vi "p4.3.vi"() -> ()   [LabVIEW 2020]
uses:
  <vilib>/Analysis/2dsp.llb/Upsample (DBL).vi
  <vilib>/Analysis/NI_AALBase.lvlib
  <vilib>/Analysis/NI_AALPro.lvlib
panel:
  out "FFT(Expansor L=3)":dbl[](graph)
  out "FFT(Expansor L=2)":dbl[](graph)
  out "FFT(original)":dbl[](graph)
  in  "L =3":i32=1
  out "Expansor L=3":dbl[](graph)
  out "Expansor L=2":dbl[](graph)
  in  "L=2":i32=1
  out "cos(0,0.3pi) + cos(0,0.4pi) - Original":dbl[](graph)
  in  "Frecuencia cos(0,4pi)":dbl=0.0078125 format="%0.4e"
  out "cos(0,0.4pi)":dbl[](graph)
  out "cos(0,0.3pi)":dbl[](graph)
  in  "Frecuencia cos(0,3pi)":dbl=0.0078125 format="%0.4e"
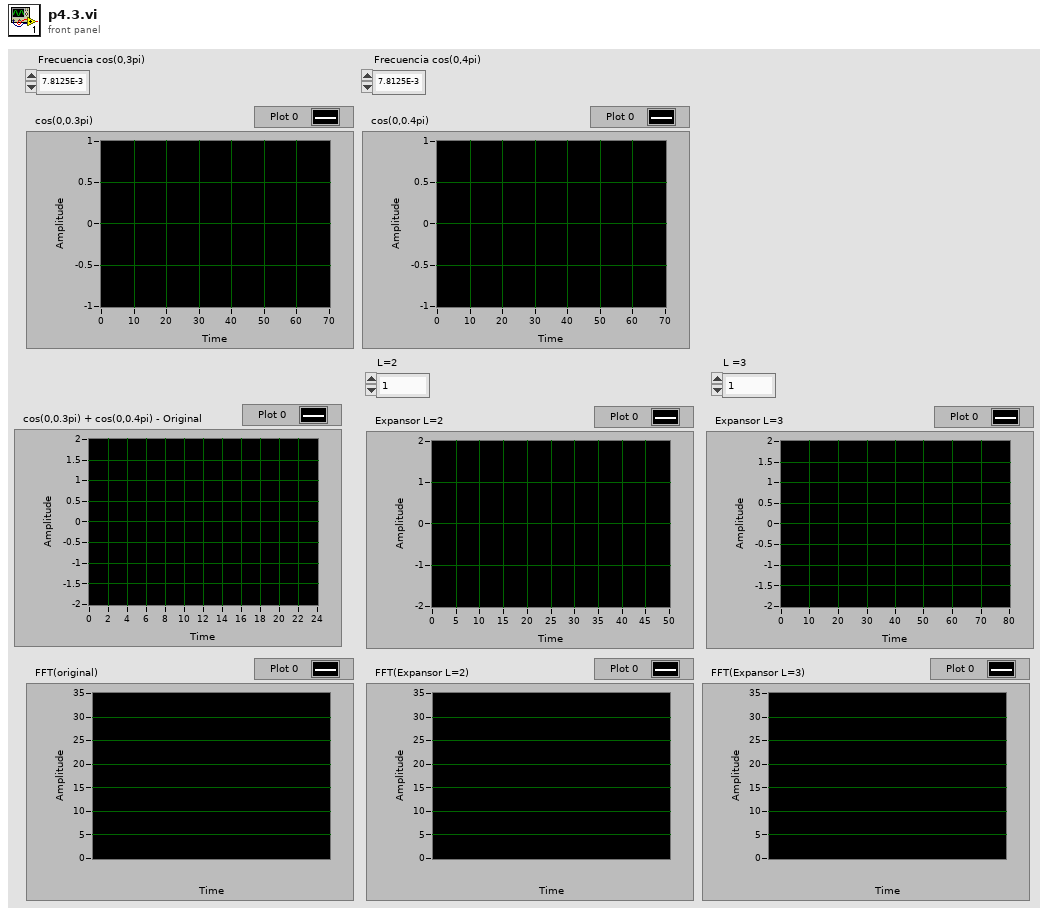
[diagram p1: front panel]
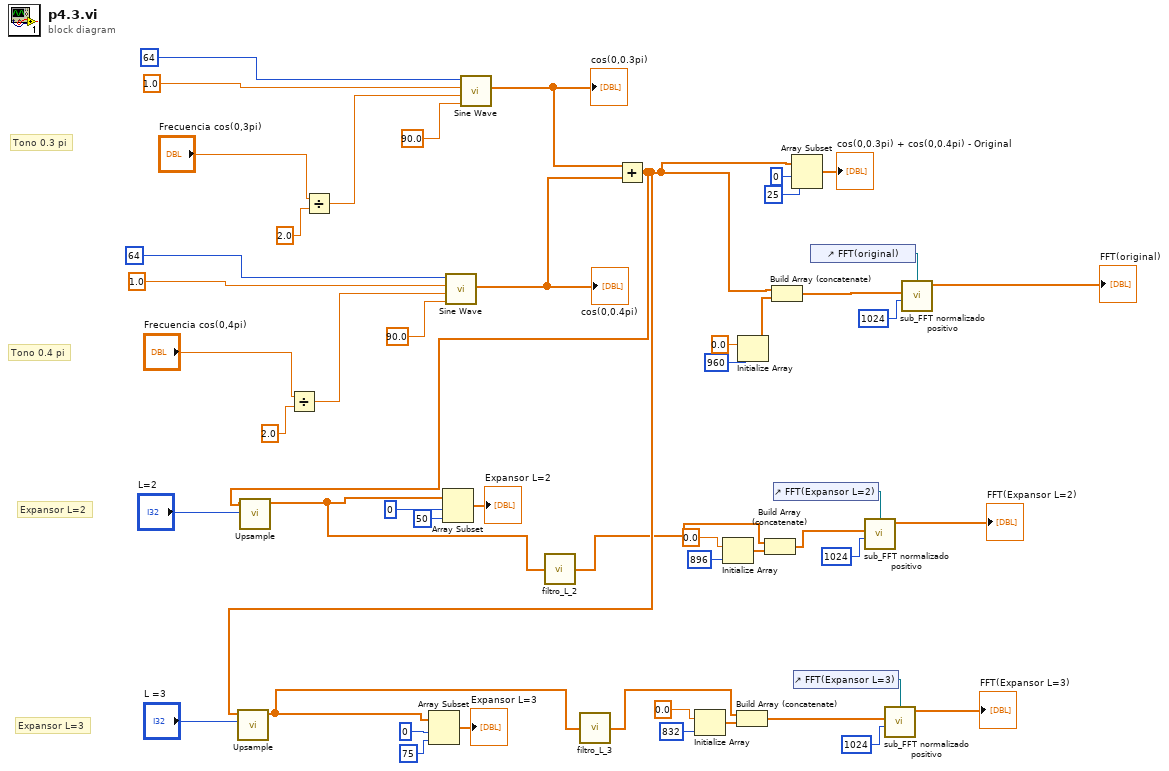
[diagram p0: block diagram]
diagram:
  # "Expansor L=3"
  # "Expansor L=2"
  # "Tono 0.4 pi"
  # "Tono 0.3 pi"
  n1 = Divide(x="Frecuencia cos(0,4pi)", y=2.0) -> (x/y=w44:dbl)
  n2 = Divide(x="Frecuencia cos(0,3pi)", y=2.0) -> (x/y=w47:dbl)
  n3 = call <vilib>:"Sine Wave.vi"("samples"=64, "amplitude"=1.0, "frequency"=w44, "phase in"=90.0) -> ("sine wave"=w38:dbl[])  [unwired: 1 in, 2 out]
  "cos(0,0.4pi)" <- w38
  n4 = call <vilib>:"Sine Wave.vi"("samples"=64, "amplitude"=1.0, "frequency"=w47, "phase in"=90.0) -> ("sine wave"=w39:dbl[])  [unwired: 1 in, 2 out]
  "cos(0,0.3pi)" <- w39
  n5 = Add(x=w39, y=w38) -> (x+y=w14:dbl[])
  n6 = call-poly <vilib>:"Upsample.vi"("upsampling factor"="L =3", "X"=w14) -> ("Upsampled Array"=w2:dbl[])  [unwired: 8 in, 1 out]
  n7 = call-poly <vilib>:"Upsample.vi"("upsampling factor"="L=2", "X"=w14) -> ("Upsampled Array"=w4:dbl[])  [unwired: 8 in, 1 out]
  n8 = Array Subset(array=w2, index=0, length=75) -> (→"Expansor L=3":dbl[])
  n9 = Array Subset(array=w4, index=0, length=50) -> (→"Expansor L=2":dbl[])
  n10 = call "filtro_L_2.vi"("x"=w4) -> ("y"=w3:dbl[])
  n11 = call "filtro_L_3.vi"("x"=w2) -> ("y"=w1:dbl[])
  n12 = Initialize Array(0.0 ("element"), 832 ("dimension size")) -> (w6:dbl[])
  n13 = Initialize Array(0.0 ("element"), 896 ("dimension size")) -> (w12:dbl[])
  n14 = Build Array (concatenate)(w1, w6) -> (w5:dbl[])
  n15 = Initialize Array(0.0 ("element"), 960 ("dimension size")) -> (w24:dbl[])
  n16 = Build Array (concatenate)(w3, w12) -> (w9:dbl[])
  n17 = Build Array (concatenate)(w14, w24) -> (w23:dbl[])
  n18 = control-ref of="FFT(Expansor L=2)"() -> (w21:refnum<vi>)
  n19 = Array Subset(array=w14, index=0, length=25) -> (→"cos(0,0.3pi) + cos(0,0.4pi) - Original":dbl[])
  n20 = control-ref of="FFT(Expansor L=3)"() -> (w16:refnum<vi>)
  n21 = control-ref of="FFT(original)"() -> (w22:refnum<vi>)
  n22 = call "sub_FFT normalizado positivo.vi"("FFT size"=1024, "Array in"=w9, "WaveformGraph in"=w21) -> ("Array out"=→"FFT(Expansor L=2)":dbl[])  [unwired: 8 in]
  n23 = call "sub_FFT normalizado positivo.vi"("FFT size"=1024, "Array in"=w5, "WaveformGraph in"=w16) -> ("Array out"=→"FFT(Expansor L=3)":dbl[])  [unwired: 8 in]
  n24 = call "sub_FFT normalizado positivo.vi"("FFT size"=1024, "Array in"=w23, "WaveformGraph in"=w22) -> ("Array out"=→"FFT(original)":dbl[])  [unwired: 8 in]
